vi "MGCC_PVFcst_EPBtest.vi"() -> ()   [LabVIEW 2016]
uses:
  Sub-VIs/f_MGCC_PVFcst_ActualPV.vi
  Active and reactvie power balance(Mark)/Labview model/Sub VIs/MGCC_PQBal_Globals.vi
  Communication (Yiwei)/Global communication.vi
  Communication (Yiwei)/Global communication output.vi
  <vilib>/Utility/error.llb/Error Cluster From Error Code.vi
  <vilib>/ErrorRing/Error Ring.xnode
  <vilib>/Analysis/NI_AALBase.lvlib
panel:
  out "f_MGCC_PVFcst_HistoricalPV 2":dbl[](graph)
  out "coerced(x) 2":dbl[](graph)
  out "f_MGCC_PVFcst_HistoricalPV":dbl[](graph)
  out "coerced(x)":dbl[](graph)
  out "error1":errorcluster
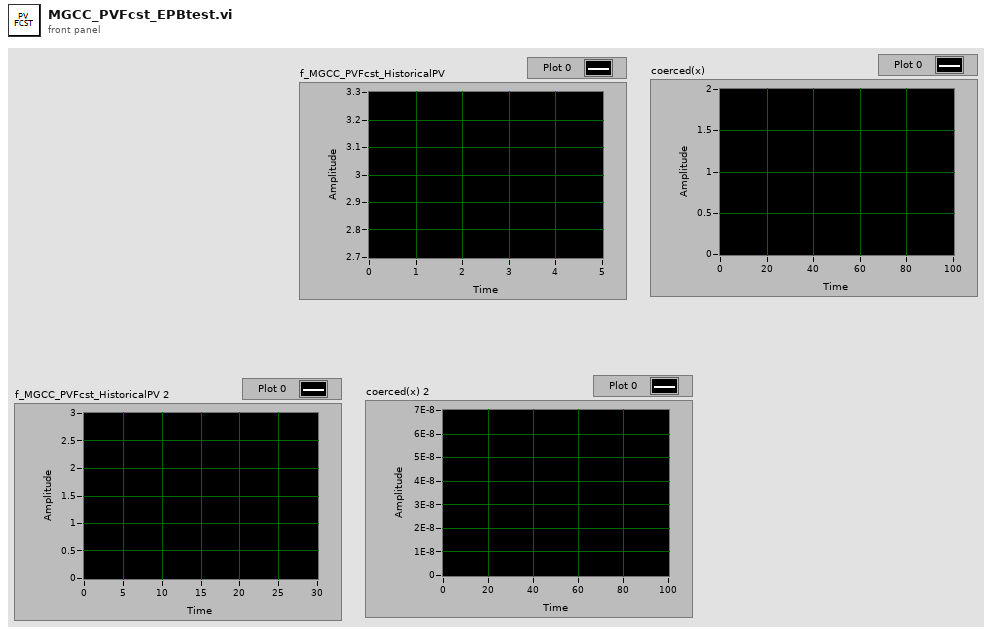
[diagram p1: front panel]
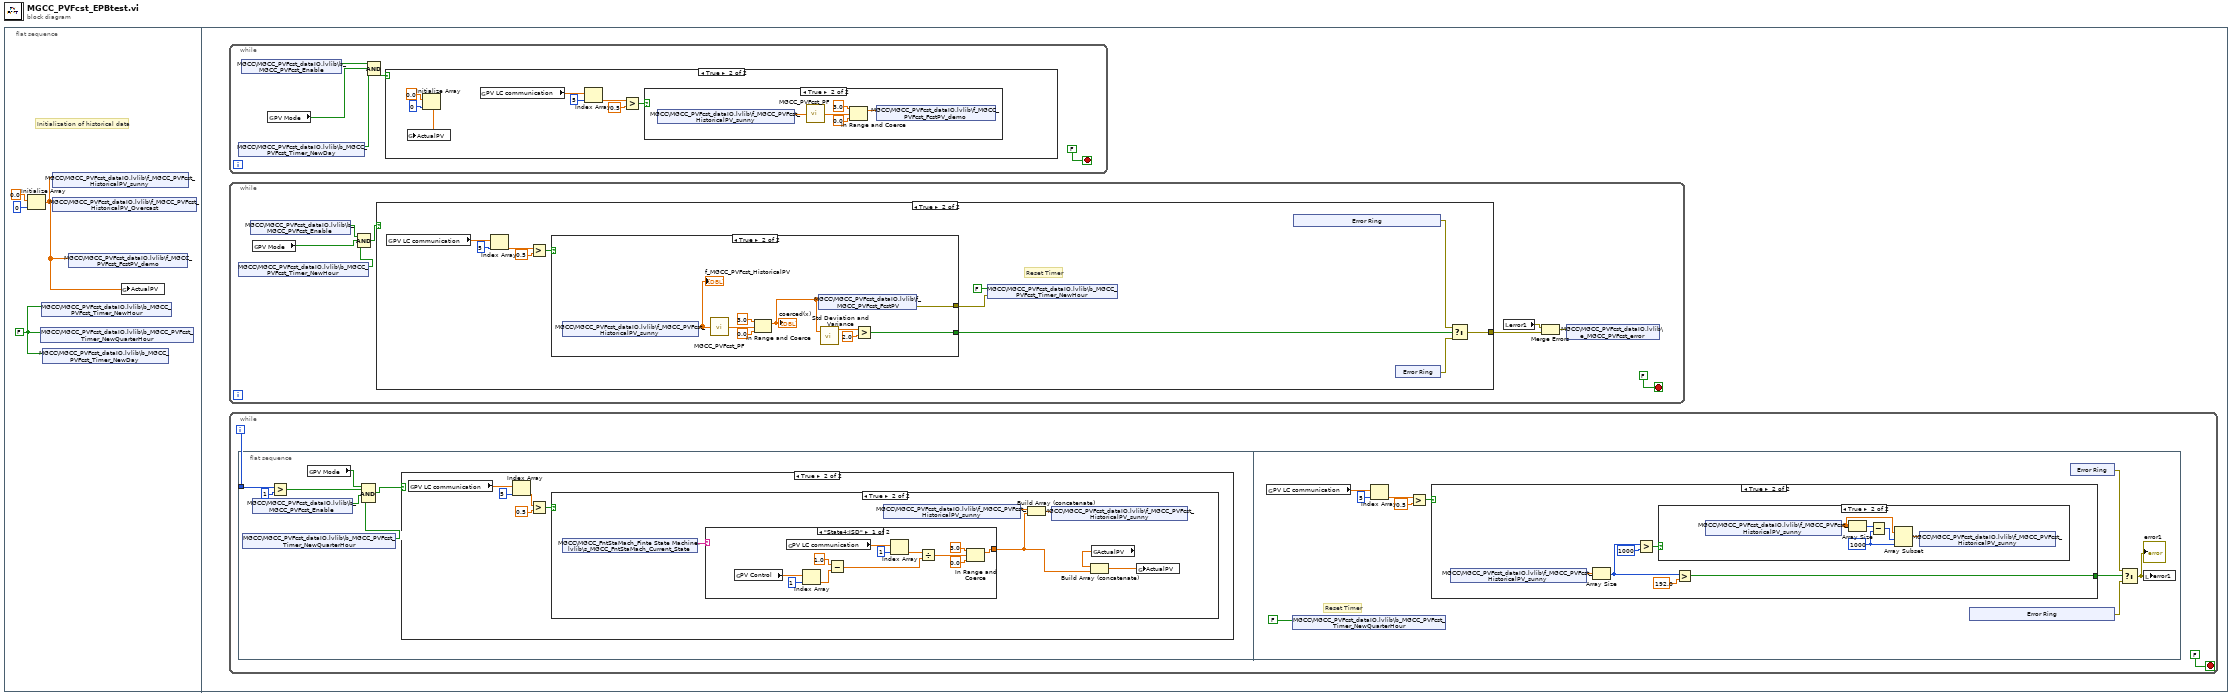
[diagram p0: block diagram]
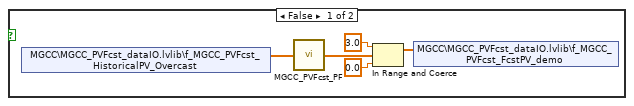
[diagram p3: hidden frame]
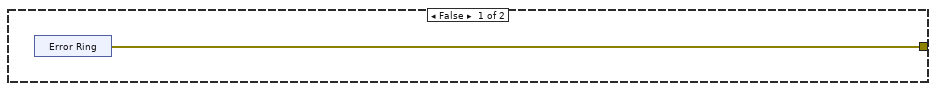
[diagram p4: hidden frame]
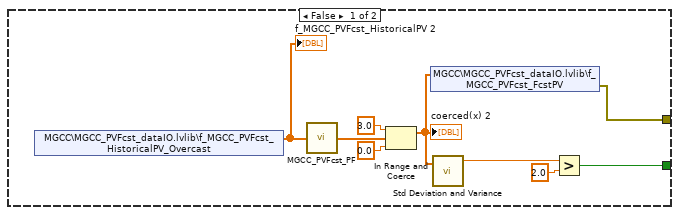
[diagram p5: hidden frame]
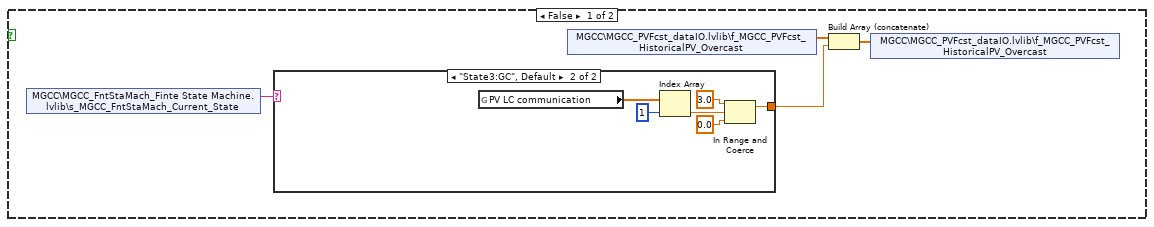
[diagram p7: hidden frame]
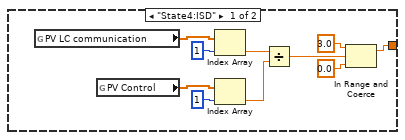
[diagram p8: hidden frame]
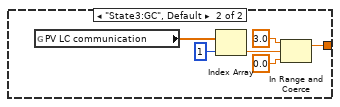
[diagram p9: hidden frame]
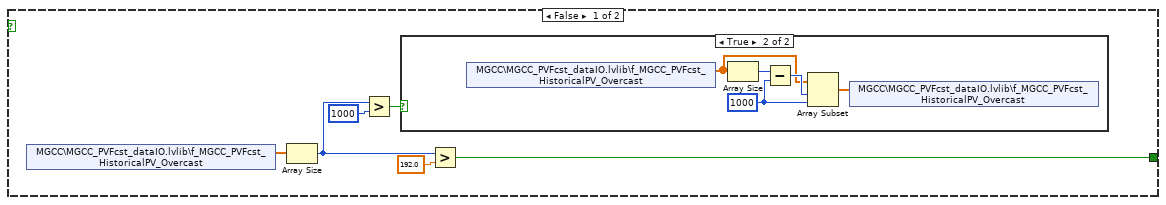
[diagram p10: hidden frame]
diagram:
  n1 = flat-sequence {
    frame #0 {
      w1 = FALSE
      # "Initialization of historical data"
      n2 = Initialize Array(0.0 ("element"), 0 ("dimension size")) -> (w2:dbl[])
      n3 = shared-variable "MGCC\\MGCC_PVFcst_dataIO.lvlib\\b_MGCC_PVFcst_Timer_NewQuarterHour"(w1) -> ()  [unwired: 1 in, 1 out]
      n4 = shared-variable "MGCC\\MGCC_PVFcst_dataIO.lvlib\\b_MGCC_PVFcst_Timer_NewHour"(w1) -> ()  [unwired: 1 in, 1 out]
      n5 = shared-variable "MGCC\\MGCC_PVFcst_dataIO.lvlib\\b_MGCC_PVFcst_Timer_NewDay"(w1) -> ()  [unwired: 1 in, 1 out]
      n6 = shared-variable "MGCC\\MGCC_PVFcst_dataIO.lvlib\\f_MGCC_PVFcst_HistoricalPV_sunny"(w2) -> ()  [unwired: 1 in, 1 out]
      n7 = shared-variable "MGCC\\MGCC_PVFcst_dataIO.lvlib\\f_MGCC_PVFcst_HistoricalPV_Overcast"(w2) -> ()  [unwired: 1 in, 1 out]
      n8 = shared-variable "MGCC\\MGCC_PVFcst_dataIO.lvlib\\f_MGCC_PVFcst_FcstPV_demo"(w2) -> ()  [unwired: 1 in, 1 out]
      n9 = global write "f_MGCC_PVFcst_ActualPV.vi" "ActualPV"(w2) -> ()
    }
    frame #1 {
      n10 = while {
        stop <- FALSE stop-if-true
        n11 = shared-variable "MGCC\\MGCC_PVFcst_dataIO.lvlib\\b_MGCC_PVFcst_Timer_NewDay"() -> (w5:bool)  [unwired: 1 in, 1 out]
        n12 = shared-variable "MGCC\\MGCC_PVFcst_dataIO.lvlib\\b_MGCC_PVFcst_Enable"() -> (w7:bool)  [unwired: 1 in, 1 out]
        n13 = global read "MGCC_PQBal_Globals.vi" "PV Mode"() -> (w6:bool)
        n14 = Compound Arithmetic op=AND(w7, w6, w5) -> (w8:bool)
        n15 = case shown="True" w8 {
          frame False {
          }
          frame True {
            n16 = Initialize Array(0.0 ("element"), 0 ("dimension size")) -> (w17:dbl[])
            n17 = global write "f_MGCC_PVFcst_ActualPV.vi" "ActualPV"(w17) -> ()
            n18 = global read "Global communication.vi" "PV LC communication"() -> (w14:dbl[])
            n19 = Index Array(array=w14, index=5) -> (element=w12:dbl)
            n20 = Greater?(x=w12, y=0.5) -> (0:w10:bool)
            n21 = case shown="True" w10 {
              frame False {
                n22 = shared-variable "MGCC\\MGCC_PVFcst_dataIO.lvlib\\f_MGCC_PVFcst_HistoricalPV_Overcast"() -> (w18:dbl[])  [unwired: 1 in, 1 out]
                n23 = call "MGCC_PVFcst_PF.vi"("InputTimeSeries"=w18) -> ("predicted series"=w21:dbl[])
                n24 = In Range and Coerce(upper limit=3.0, x=w21, lower limit=0.0) -> (coerced(x)=w22:dbl[])  [unwired: 1 out]
                n25 = shared-variable "MGCC\\MGCC_PVFcst_dataIO.lvlib\\f_MGCC_PVFcst_FcstPV_demo"(w22) -> ()  [unwired: 1 in, 1 out]
              }
              frame True {
                n26 = shared-variable "MGCC\\MGCC_PVFcst_dataIO.lvlib\\f_MGCC_PVFcst_HistoricalPV_sunny"() -> (w27:dbl[])  [unwired: 1 in, 1 out]
                n27 = call "MGCC_PVFcst_PF.vi"("InputTimeSeries"=w27) -> ("predicted series"=w24:dbl[])
                n28 = In Range and Coerce(upper limit=3.0, x=w24, lower limit=0.0) -> (coerced(x)=w23:dbl[])  [unwired: 1 out]
                n29 = shared-variable "MGCC\\MGCC_PVFcst_dataIO.lvlib\\f_MGCC_PVFcst_FcstPV_demo"(w23) -> ()  [unwired: 1 in, 1 out]
              }
            }
          }
        }
      }
      n30 = while {
        stop <- FALSE stop-if-true
        n31 = shared-variable "MGCC\\MGCC_PVFcst_dataIO.lvlib\\b_MGCC_PVFcst_Timer_NewHour"() -> (w29:bool)  [unwired: 1 in, 1 out]
        n32 = shared-variable "MGCC\\MGCC_PVFcst_dataIO.lvlib\\b_MGCC_PVFcst_Enable"() -> (w31:bool)  [unwired: 1 in, 1 out]
        n33 = global read "MGCC_PQBal_Globals.vi" "PV Mode"() -> (w30:bool)
        n34 = Compound Arithmetic op=AND(w31, w30, w29) -> (w28:bool)
        n35 = case shown="True" w28 {
          tunnel: [w36 w45] -> w34
          frame False {
            n36 = xnode "Error Ring"() -> ("error out"=w36:errorcluster)
          }
          frame True {
            # "Reset Timer"
            n37 = global read "Global communication.vi" "PV LC communication"() -> (w44:dbl[])
            n38 = Index Array(array=w44, index=5) -> (element=w42:dbl)
            n39 = Greater?(x=w42, y=0.5) -> (0:w40:bool)
            n40 = case shown="True" w40 {
              tunnel: [w50 w59] -> w46
              tunnel: [w49 w58] -> w38
              frame False {
                n41 = shared-variable "MGCC\\MGCC_PVFcst_dataIO.lvlib\\f_MGCC_PVFcst_HistoricalPV_Overcast"() -> (w51:dbl[])  [unwired: 1 in, 1 out]
                "f_MGCC_PVFcst_HistoricalPV 2" <- w51
                n42 = call "MGCC_PVFcst_PF.vi"("InputTimeSeries"=w51) -> ("predicted series"=w54:dbl[])
                n43 = In Range and Coerce(upper limit=3.0, x=w54, lower limit=0.0) -> (coerced(x)=w57:dbl[])  [unwired: 1 out]
                "coerced(x) 2" <- w57
                n44 = shared-variable "MGCC\\MGCC_PVFcst_dataIO.lvlib\\f_MGCC_PVFcst_FcstPV"(w57) -> (error out=w49:errorcluster)  [unwired: 1 in]
                n45 = call <vilib>:"Std Deviation and Variance.vi"("X"=w57) -> ("mean"=w56:dbl)  [unwired: 1 in, 2 out]
                n46 = Greater?(x=w56, y=2.0) -> (0:w50:bool)
              }
              frame True {
                n47 = shared-variable "MGCC\\MGCC_PVFcst_dataIO.lvlib\\f_MGCC_PVFcst_HistoricalPV_sunny"() -> (w66:dbl[])  [unwired: 1 in, 1 out]
                "f_MGCC_PVFcst_HistoricalPV" <- w66
                n48 = call "MGCC_PVFcst_PF.vi"("InputTimeSeries"=w66) -> ("predicted series"=w63:dbl[])
                n49 = In Range and Coerce(upper limit=3.0, x=w63, lower limit=0.0) -> (coerced(x)=w60:dbl[])  [unwired: 1 out]
                "coerced(x)" <- w60
                n50 = shared-variable "MGCC\\MGCC_PVFcst_dataIO.lvlib\\f_MGCC_PVFcst_FcstPV"(w60) -> (error out=w58:errorcluster)  [unwired: 1 in]
                n51 = call <vilib>:"Std Deviation and Variance.vi"("X"=w60) -> ("mean"=w61:dbl)  [unwired: 1 in, 2 out]
                n52 = Greater?(x=w61, y=2.0) -> (0:w59:bool)
              }
            }
            n53 = shared-variable "MGCC\\MGCC_PVFcst_dataIO.lvlib\\b_MGCC_PVFcst_Timer_NewHour"(FALSE ("b_MGCC_PVFcst_Timer_NewHour"), error in=w38) -> ()  [unwired: 1 out]
            n54 = xnode "Error Ring"() -> ("error out"=w48:errorcluster)
            n55 = xnode "Error Ring"() -> ("error out"=w47:errorcluster)
            n56 = Select(t=w48, s=w46, f=w47) -> (s? t:f=w45:errorcluster)
          }
        }
        n57 = local read "error1"() -> (w32:errorcluster)
        n58 = Merge Errors(w32, w34) -> (w33:errorcluster)
        n59 = shared-variable "MGCC\\MGCC_PVFcst_dataIO.lvlib\\e_MGCC_PVFcst_error"(w33) -> ()  [unwired: 1 in, 1 out]
      }
      n60 = while {
        i -> [w73]
        stop <- FALSE stop-if-true
        n61 = flat-sequence {
          tunnel: w73 -> [w80]
          frame #0 {
            n62 = shared-variable "MGCC\\MGCC_PVFcst_dataIO.lvlib\\b_MGCC_PVFcst_Timer_NewQuarterHour"() -> (w75:bool)  [unwired: 1 in, 1 out]
            n63 = shared-variable "MGCC\\MGCC_PVFcst_dataIO.lvlib\\b_MGCC_PVFcst_Enable"() -> (w76:bool)  [unwired: 1 in, 1 out]
            n64 = Greater?(x=w80, y=1) -> (0:w77:bool)
            n65 = global read "MGCC_PQBal_Globals.vi" "PV Mode"() -> (w78:bool)
            n66 = Compound Arithmetic op=AND(w78, w77, w76, w75) -> (w79:bool)
            n67 = case shown="True" w79 {
              frame False {
              }
              frame True {
                n68 = global read "Global communication.vi" "PV LC communication"() -> (w86:dbl[])
                n69 = Index Array(array=w86, index=5) -> (element=w84:dbl)
                n70 = Greater?(x=w84, y=0.5) -> (0:w82:bool)
                n71 = case shown="True" w82 {
                  frame False {
                    n72 = shared-variable "MGCC\\MGCC_FntStaMach_Finte State Machine.lvlib\\s_MGCC_FntStaMach_Current_State"() -> (w87:string)  [unwired: 1 in, 1 out]
                    n73 = case shown="\"State3:GC\", Default" w87 {
                      tunnel: [w91 w104] -> w88
                      frame "State4:ISD" {
                        n74 = global read "Global communication.vi" "PV LC communication"() -> (w98:dbl[])
                        n75 = global read "Global communication output.vi" "PV Control"() -> (w95:dbl[])
                        n76 = Index Array(array=w98, index=1) -> (element=w92:dbl)
                        n77 = Index Array(array=w95, index=1) -> (element=w94:dbl)
                        n78 = Divide(x=w92, y=w94) -> (x/y=w93:dbl)
                        n79 = In Range and Coerce(upper limit=3.0, x=w93, lower limit=0.0) -> (coerced(x)=w91:dbl)  [unwired: 1 out]
                      }
                      frame "State3:GC", Default {
                        n80 = global read "Global communication.vi" "PV LC communication"() -> (w103:dbl[])
                        n81 = Index Array(array=w103, index=1) -> (element=w101:dbl)
                        n82 = In Range and Coerce(upper limit=3.0, x=w101, lower limit=0.0) -> (coerced(x)=w104:dbl)  [unwired: 1 out]
                      }
                    }
                    n83 = shared-variable "MGCC\\MGCC_PVFcst_dataIO.lvlib\\f_MGCC_PVFcst_HistoricalPV_Overcast"() -> (w90:dbl[])  [unwired: 1 in, 1 out]
                    n84 = Build Array (concatenate)(w90, w88) -> (w89:dbl[])
                    n85 = shared-variable "MGCC\\MGCC_PVFcst_dataIO.lvlib\\f_MGCC_PVFcst_HistoricalPV_Overcast"(w89) -> ()  [unwired: 1 in, 1 out]
                  }
                  frame True {
                    n86 = shared-variable "MGCC\\MGCC_FntStaMach_Finte State Machine.lvlib\\s_MGCC_FntStaMach_Current_State"() -> (w110:string)  [unwired: 1 in, 1 out]
                    n87 = case shown="\"State4:ISD\"" w110 {
                      tunnel: [w116 w128] -> w107
                      frame "State4:ISD" {
                        n88 = global read "Global communication output.vi" "PV Control"() -> (w119:dbl[])
                        n89 = global read "Global communication.vi" "PV LC communication"() -> (w122:dbl[])
                        n90 = Index Array(array=w119, index=1) -> (element=w115:dbl)
                        n91 = Subtract(x=1.0, y=w115) -> (x-y=w113:dbl)
                        n92 = Index Array(array=w122, index=1) -> (element=w117:dbl)
                        n93 = Divide(x=w117, y=w113) -> (x/y=w118:dbl)
                        n94 = In Range and Coerce(upper limit=3.0, x=w118, lower limit=0.0) -> (coerced(x)=w116:dbl)  [unwired: 1 out]
                      }
                      frame "State3:GC", Default {
                        n95 = global read "Global communication.vi" "PV LC communication"() -> (w127:dbl[])
                        n96 = Index Array(array=w127, index=1) -> (element=w125:dbl)
                        n97 = In Range and Coerce(upper limit=3.0, x=w125, lower limit=0.0) -> (coerced(x)=w128:dbl)  [unwired: 1 out]
                      }
                    }
                    n98 = shared-variable "MGCC\\MGCC_PVFcst_dataIO.lvlib\\f_MGCC_PVFcst_HistoricalPV_sunny"() -> (w112:dbl[])  [unwired: 1 in, 1 out]
                    n99 = Build Array (concatenate)(w112, w107) -> (w111:dbl[])
                    n100 = shared-variable "MGCC\\MGCC_PVFcst_dataIO.lvlib\\f_MGCC_PVFcst_HistoricalPV_sunny"(w111) -> ()  [unwired: 1 in, 1 out]
                    n101 = global read "f_MGCC_PVFcst_ActualPV.vi" "ActualPV"() -> (w108:dbl[])
                    n102 = Build Array (concatenate)(w108, w107) -> (w109:dbl[])
                    n103 = global write "f_MGCC_PVFcst_ActualPV.vi" "ActualPV"(w109) -> ()
                  }
                }
              }
            }
          }
          frame #1 {
            # "Reset Timer"
            n104 = global read "Global communication.vi" "PV LC communication"() -> (w136:dbl[])
            n105 = shared-variable "MGCC\\MGCC_PVFcst_dataIO.lvlib\\b_MGCC_PVFcst_Timer_NewQuarterHour"(FALSE) -> ()  [unwired: 1 in, 1 out]
            n106 = Index Array(array=w136, index=5) -> (element=w134:dbl)
            n107 = Greater?(x=w134, y=0.5) -> (0:w132:bool)
            n108 = case shown="True" w132 {
              tunnel: [w142 w152] -> w138
              frame False {
                n109 = shared-variable "MGCC\\MGCC_PVFcst_dataIO.lvlib\\f_MGCC_PVFcst_HistoricalPV_Overcast"() -> (w143:dbl[])  [unwired: 1 in, 1 out]
                n110 = Array Size(array=w143) -> (size(s)=w146:i32)
                n111 = Greater?(x=w146, y=1000) -> (0:w141:bool)
                n112 = case shown="True" w141 {
                  frame False {
                  }
                  frame True {
                    w151 = 1000 ("y")
                    n113 = shared-variable "MGCC\\MGCC_PVFcst_dataIO.lvlib\\f_MGCC_PVFcst_HistoricalPV_Overcast"() -> (w147:dbl[])  [unwired: 1 in, 1 out]
                    n114 = Array Size(array=w147) -> (size(s)=w148:i32)
                    n115 = Subtract(x=w148, y=w151) -> (x-y=w149:i32)
                    n116 = Array Subset(array=w147, index=w149, length=w151) -> (w150:dbl[])
                    n117 = shared-variable "MGCC\\MGCC_PVFcst_dataIO.lvlib\\f_MGCC_PVFcst_HistoricalPV_Overcast"(w150) -> ()  [unwired: 1 in, 1 out]
                  }
                }
                n118 = Greater?(x=w146, y=192.0) -> (0:w142:bool)
              }
              frame True {
                n119 = shared-variable "MGCC\\MGCC_PVFcst_dataIO.lvlib\\f_MGCC_PVFcst_HistoricalPV_sunny"() -> (w157:dbl[])  [unwired: 1 in, 1 out]
                n120 = Array Size(array=w157) -> (size(s)=w153:i32)
                n121 = Greater?(x=w153, y=1000) -> (0:w155:bool)
                n122 = case shown="True" w155 {
                  frame False {
                  }
                  frame True {
                    w158 = 1000 ("y")
                    n123 = shared-variable "MGCC\\MGCC_PVFcst_dataIO.lvlib\\f_MGCC_PVFcst_HistoricalPV_sunny"() -> (w162:dbl[])  [unwired: 1 in, 1 out]
                    n124 = Array Size(array=w162) -> (size(s)=w161:i32)
                    n125 = Subtract(x=w161, y=w158) -> (x-y=w160:i32)
                    n126 = Array Subset(array=w162, index=w160, length=w158) -> (w159:dbl[])
                    n127 = shared-variable "MGCC\\MGCC_PVFcst_dataIO.lvlib\\f_MGCC_PVFcst_HistoricalPV_sunny"(w159) -> ()  [unwired: 1 in, 1 out]
                  }
                }
                n128 = Greater?(x=w153, y=192.0) -> (0:w152:bool)
              }
            }
            n129 = xnode "Error Ring"() -> ("error out"=w139:errorcluster)
            n130 = xnode "Error Ring"() -> ("error out"=w140:errorcluster)
            n131 = Select(t=w140, s=w138, f=w139) -> (s? t:f=w137:errorcluster)
            "error1" <- w137
            n132 = local write "error1"(w137) -> ()
          }
        }
      }
    }
  }
